vi "Position actual value.vi"(8 "error in":errorcluster, 11 "Motor Base in":refnum<class "Motor Base.lvclass">) -> (0 "error out":errorcluster, 2 "Data":i32, 3 "Motor Base out":refnum<class "Motor Base.lvclass">)   [LabVIEW 2016, in "Motor Base.lvlib" / "Motor Base.lvclass"]
uses:
  Motor Base.lvclass
  Data Type.ctl
  AccessType.ctl
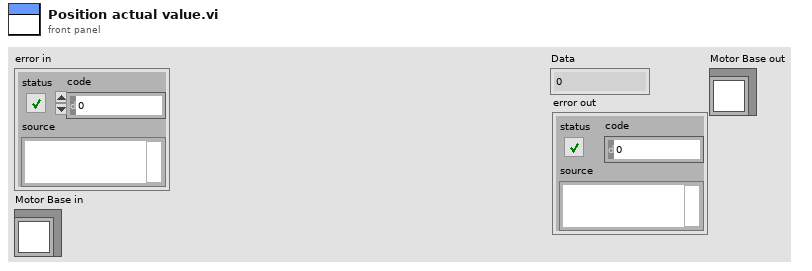
[diagram p1: front panel]
types:
  T1 = typedef "Motor Base.lvlib/Motor Base.lvclass/AccessType.ctl" = enum16{"Write", "Read", "Read Only"}
  T2 = typedef "Motor Base.lvlib/Motor Base.lvclass/Data Type.ctl" = enum16{"BOOL", "I16", "I32", "I8", "OS", "U16", "U32", "U8", "VS"}
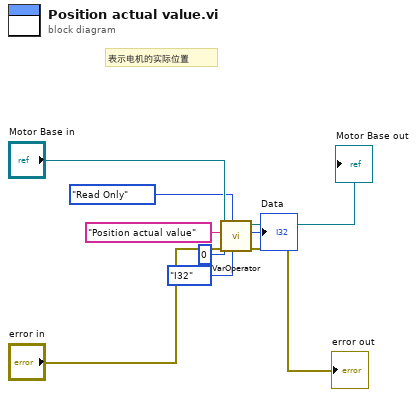
[diagram p0: block diagram]
diagram:
  # "表示电机的实际位置"
  n1 = call-dynamic "VarOperator.vi"("Data Type"=Data_Type."I32", "ro/w/r"=AccessType."Read Only", "error in"="error in", "Data"=i64 0, "PDO Name"="Position actual value", "Motor Base in"="Motor Base in") -> ("error out"=→"error out":errorcluster, "Data"=→"Data":i64, "Motor Base out"=→"Motor Base out":refnum<class "Motor Base.lvclass">)  [unwired: 1 in, 2 out]
